vi "Cheby 2D array prep_XY spreadsheet.vi"(7 "end":dbl=7.0 format="%.2f", 8 "start":dbl format="%.2f", 9 "order":u32=14, 10 "spreadsheet string":string) -> (2 "original curve":cluster{dbl[], dbl[]}, 3 "values":dbl[](array[numeric]))   [LabVIEW 2021]
panel:
  out "output cluster":cluster{dbl[], dbl[]}
  out "XY Graph":cluster{dbl[], dbl[]}[](graph)
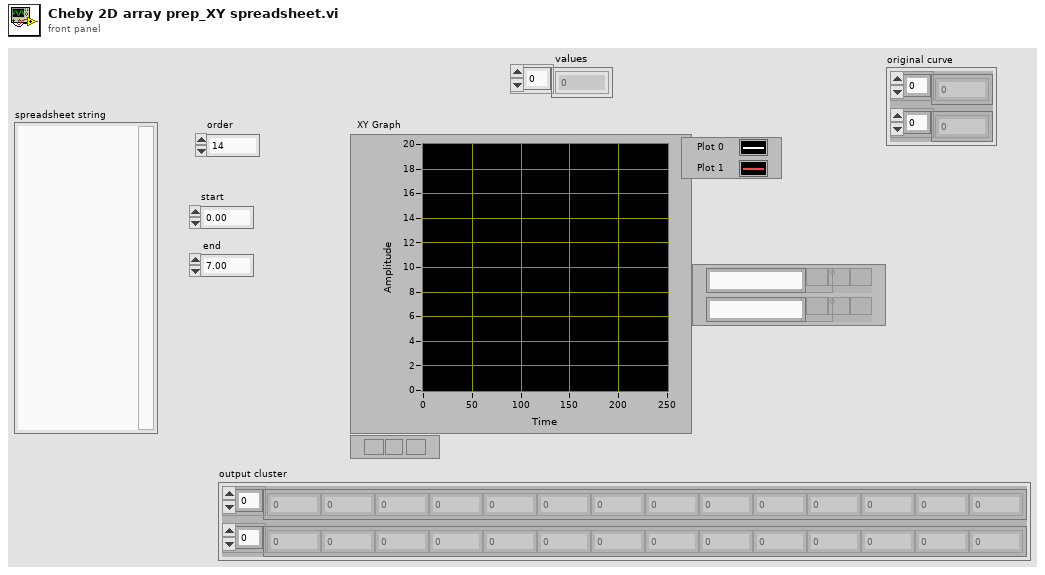
[diagram p1: front panel]
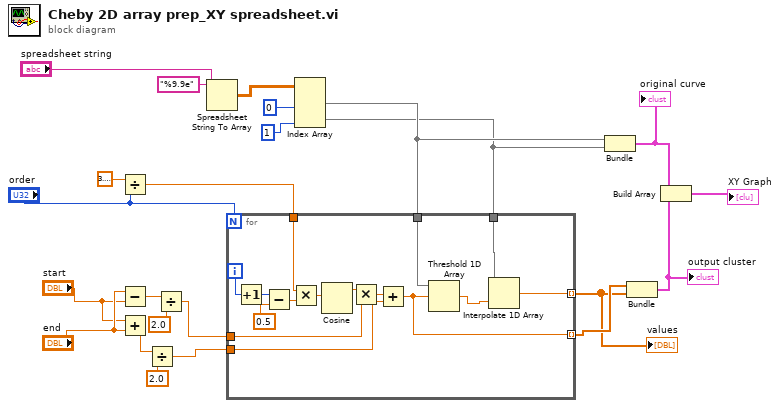
[diagram p0: block diagram]
diagram:
  n1 = Divide(x=3.141592653589793, y="order") -> (x/y=w13:dbl)
  n2 = Subtract(x="end", y="start") -> (x-y=w18:dbl)
  n3 = Add(x="start", y="end") -> (x+y=w20:dbl)
  n4 = Divide(x=w20, y=2.0) -> (x/y=w15:dbl)
  n5 = Divide(x=w18, y=2.0) -> (x/y=w16:dbl)
  n6 = Spreadsheet String To Array(format string="%9.9e", spreadsheet string="spreadsheet string") -> (array=w1:dbl[][])  [unwired: 2 in]
  n7 = Index Array(array=w1, index (col) #1=0 ("disabled index (col)"), index (col) #2=1 ("index (col)")) -> (element #1=w10:dbl[], element #2=w9:dbl[])  [unwired: 2 in]
  n8 = for {
    N: "order" -> [_]
    tunnel: w13 -> [w36]
    tunnel: w16 -> [w32]
    tunnel: w15 -> [w29]
    tunnel: w10 -> [w28]
    tunnel: w9 -> [w27]
    tunnel: [w25] -> w2 mode=indexing
    tunnel: [w24] -> w3 mode=indexing
    i -> [w37]
    n9 = Increment(x=w37) -> (x+1=w33:i32)
    n10 = Subtract(x=w33, y=0.5) -> (x-y=w35:dbl)
    n11 = Multiply(x=w36, y=w35) -> (x*y=w34:dbl)
    n12 = Cosine(x=w34) -> (cos(x)=w31:dbl)
    n13 = Multiply(x=w31, y=w32) -> (x*y=w30:dbl)
    n14 = Add(x=w30, y=w29) -> (x+y=w24:dbl)
    n15 = Threshold 1D Array(2:w24, 3:w28) -> (0:w26:dbl)  [unwired: 1 in]
    n16 = Interpolate 1D Array(1:w26, 2:w27) -> (0:w25:dbl)
  }
  "values" <- w2
  n17 = Bundle(w10, w9) -> (w7:cluster{dbl[], dbl[]})  [unwired: 1 in]
  "original curve" <- w7
  n18 = Bundle(w3, w2) -> (w8:cluster{dbl[], dbl[]})  [unwired: 1 in]
  "output cluster" <- w8
  n19 = Build Array(w7, w8) -> (→"XY Graph":cluster{dbl[], dbl[]}[])
